vi "Initialize Representation.vi"(8 "error in (no error)":errorcluster, 11 "Numeric Data Type in":refnum<class "Numeric Data Type.lvclass">) -> (0 "error out":errorcluster, 3 "Numeric Data Type (dup)":refnum<class "Numeric Data Type.lvclass">)   [LabVIEW 2018, in "Numeric Data Type.lvclass"]
uses:
  Numeric Data Type.lvclass
  Numeric Data Type.lvclass/Numeric Data Type.ctl
  Reference Representation.vi
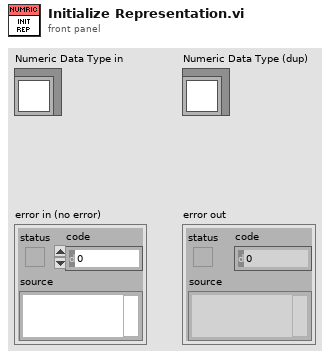
[diagram p1: front panel]
types:
  T1 = typedef "Numeric Data Type.lvclass/Representation Enum.ctl" = enum16{"Extended (EXT)", "Double (DBL)", "Single (SGL)", "Fixed-Point (FXP)", "Quad Integer (I64)", "Long Integer (I32)", "Word Integer (I16)", "Byte Integer (I8)", "Unsigned Quad (U64)", "Unsigned Long (U32)", "Unsigned Word (U16)", "Unsigned Byte (U8)", "Complex Extended (CXT)", "Complex Double (CDB)", "Complex Single (CSG)"}
  T2 = typedef "Numeric Data Type.lvclass/Representation Ring.ctl" = u16
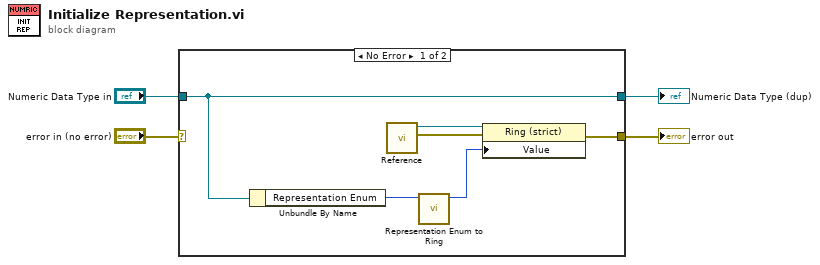
[diagram p0: block diagram]
diagram:
  n1 = case shown="No Error" "error in (no error)" {
    selector: "error in (no error)" -> [_ w12]
    tunnel: [w7 w12] -> w3
    tunnel: [w10 w11] -> w1
    tunnel: "Numeric Data Type in" -> [w10 w11]
    frame No Error {
      n2 = Unbundle By Name(w10) -> ("Representation Enum"=w9:T1)
      n3 = call-poly "Reference.vi"() -> ("error out"=w5:errorcluster, "Representation"=w6:refnum<vi>)  [unwired: 10 in]
      n4 = call "Representation Enum to Ring.vi"("Representation Enum"=w9) -> ("Representation Ring"=w8:T2)  [unwired: 10 in]
      n5 = property class="Ring (strict)"(reference=w6, error in=w5, "Value"=w8) -> (error out=w7:errorcluster)  [unwired: 1 out]
    }
    frame Error {
    }
  }
  "error out" <- w3
  "Numeric Data Type (dup)" <- w1
